vi "CleanUp.vi"(8 "error in (no error)":errorcluster, 11 "object in":refnum<class "NativeBaseTemplate_4x4x4.lvclass">) -> (0 "error out":errorcluster, 3 "object out":refnum<class "NativeBaseTemplate_4x4x4.lvclass">)   [LabVIEW 2020, in "NativeBaseTemplate_4x4x4.lvclass"]
uses:
  <resource>/Framework/Providers/Open_GDS/ClassProviders/Provider_LvNativeClass/Templates/NativeBaseTemplate_4x4x4/NativeBaseTemplate_4x4x4.lvclass
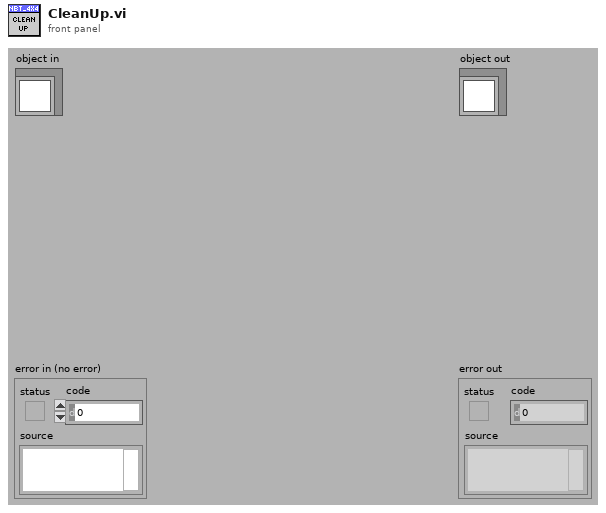
[diagram p1: front panel]
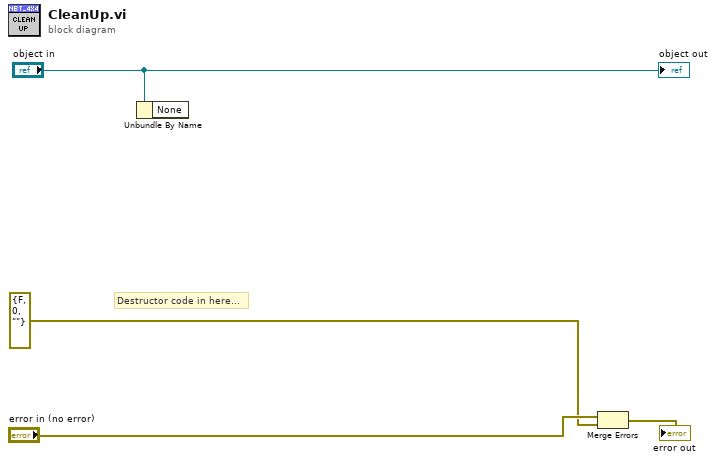
[diagram p0: block diagram]
diagram:
  # "Destructor code in here..."
  n1 = Unbundle By Name("object in") -> ()  [unwired: 1 out]
  n2 = Merge Errors("error in (no error)", errorcluster {"status"=FALSE, "code"=0, "source"=""} ("error in (no error)")) -> (→"error out":errorcluster)
  "object out" <- "object in"
